vi "PXI_Host_LargeFXP_Write_NewMethod_Benchmark.vi"() -> ()   [LabVIEW 2018]
uses:
  <vilib>/Platform/TimedLoop/XDataNode/timing_clust.ctl
  <vilib>/Platform/TimedLoop/XDataNode/nitl_modes.ctl
  <vilib>/Platform/TimedLoop/XDataNode/wakeup.ctl
  cRIO RT/FPGA Bitfile Register Operations/Scalar IO Operations/TypeDefs/FXP Configuration.ctl
  <vilib>/fxp/LVFixedPointRepBitsTypeDef.ctl
  <vilib>/fxp/LVFixedPointRepRangeTypeDef.ctl
  cRIO RT/FPGA Bitfile Register Operations/Scalar IO Operations/Write Methods/Write Data Register/Instances/Write FXP.vi
  cRIO RT/FPGA Bitfile Register Operations/Scalar IO Operations/Write Methods/Write Data Register/Instances/Write U16.vi
  cRIO RT/FPGA Bitfile Register Operations/Scalar IO Operations/Write Methods/Write Data Register/Instances/Write U32.vi
  cRIO RT/FPGA Bitfile Register Operations/Scalar IO Operations/Write Methods/Write Data Register/Instances/Write U64.vi
  cRIO RT/FPGA Bitfile Register Operations/Scalar IO Operations/Write Methods/Write Data Register/Instances/Write U8.vi
  cRIO RT/FPGA Bitfile Register Operations/Scalar IO Operations/SubVIs/DBL to FXP Raw.vi
  cRIO RT/FPGA Bitfile Register Operations/Scalar IO Operations/Utilities/Find Register Offset.vi
  cRIO RT/FPGA Bitfile Register Operations/Scalar IO Operations/SubVIs/Check Register Data Store.vi
  cRIO RT/FPGA Bitfile Register Operations/Scalar IO Operations/Error Handling/Error 6001.vi
  cRIO RT/FPGA Bitfile Register Operations/Scalar IO Operations/Error Handling/Error 6000.vi
  cRIO RT/FPGA Bitfile Register Operations/Scalar IO Operations/Error Handling/Error 6002.vi
  cRIO RT/FPGA Bitfile Register Operations/Scalar IO Operations/Error Handling/Error 6006.vi
  <vilib>/FPGAPlugInAG/Dynamic/niLvFpga_Close_Dynamic.vi
  <vilib>/platform/TimedLoop/XDataNode/XDataNode.xnode
  <vilib>/rvi/interface/nirviCloseFPGA/nirviCloseFPGA.xnode
  cRIO RT/FPGA Bitfile Register Operations/Scalar IO Operations/FPGA Register IO.lvlib
  <vilib>/Platform/TimedLoop/XDataNode/XDNodeRunTimeDep.lvlib
panel:
  out "Maximum(s)":dbl
  out "Standard deviation":dbl
  out "Waveform Graph":dbl[](graph)
  out "error out":errorcluster
  out "Execution time (s)":dbl
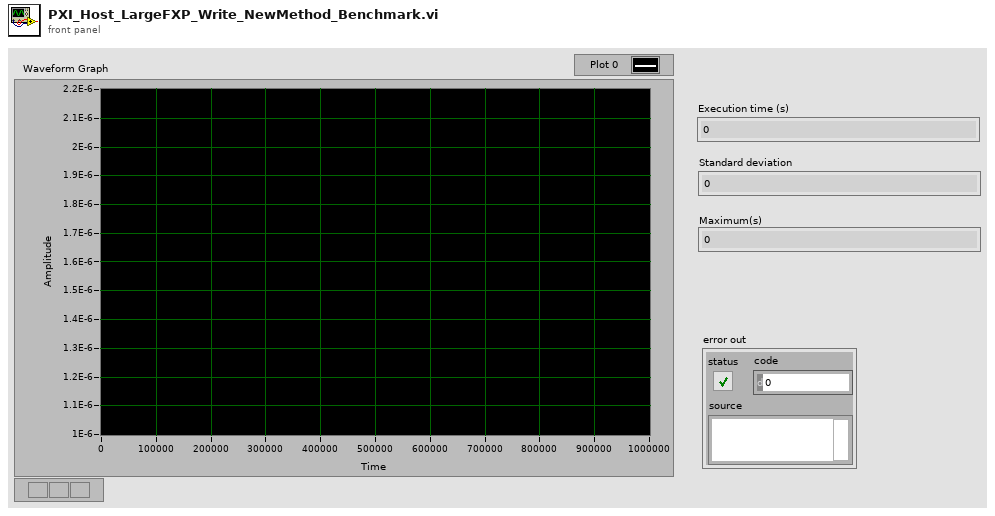
[diagram p1: front panel]
types:
  T1 = typedef "FPGA Register IO.lvlib/FXP Configuration.ctl" = cluster{"FXP Representation":T2, "FXP Range":T3}
  T2 = typedef "LVFixedPointRepBitsTypeDef.ctl" = cluster{"Signed":bool, "Word Length":u32, "Integer Word Length":i32}
  T3 = typedef "LVFixedPointRepRangeTypeDef.ctl" = cluster{"Range Min":dbl, "Range Max":dbl, "Delta":dbl}
  T4 = typedef "XDNodeRunTimeDep.lvlib/timing_clust.ctl" = cluster{"Expected End [f-1]":u64, "Actual End [f-1]":u64, "Finished Late? [f-1]":bool, "Expected End [i-1]":u64, "Actual End [i-1]":u64, "Finished Late? [i-1]":bool, "Expected Start [i]":u64, "Actual Start [i]":u64, "Expected Start [f]":u64, "Actual Start [f]":u64, "Source Name":string, "Structure Name":string, "Period":i64, "Deadline":i64, "Offset":i64, "Start":i64, "Priority":i32, "Timeout":i32, "Mode":T5, "Wakeup Reason":T6, "Error":errorcluster, "Source Type":string, "Secondary Source Type":string, "Global End Time":u64, "Global Start Time":u64, "Frame Duration":u64, "Iteration Duration":u64, "Assigned CPU":i32, "I/O Scan Engine Mode":u32}
  T5 = typedef "XDNodeRunTimeDep.lvlib/nitl_modes.ctl" = enum32{"No Change", "Process missed periods, maintain original phase", "Discard missed periods, maintain original phase", "Process missed periods, ignore original phase", "Discard missed periods, ignore original phase"}
  T6 = typedef "XDNodeRunTimeDep.lvlib/wakeup.ctl" = enum32{"Normal", "Aborted", "Asynchronous wakeup", "Timing source error", "Timed loop error", "Timeout"}
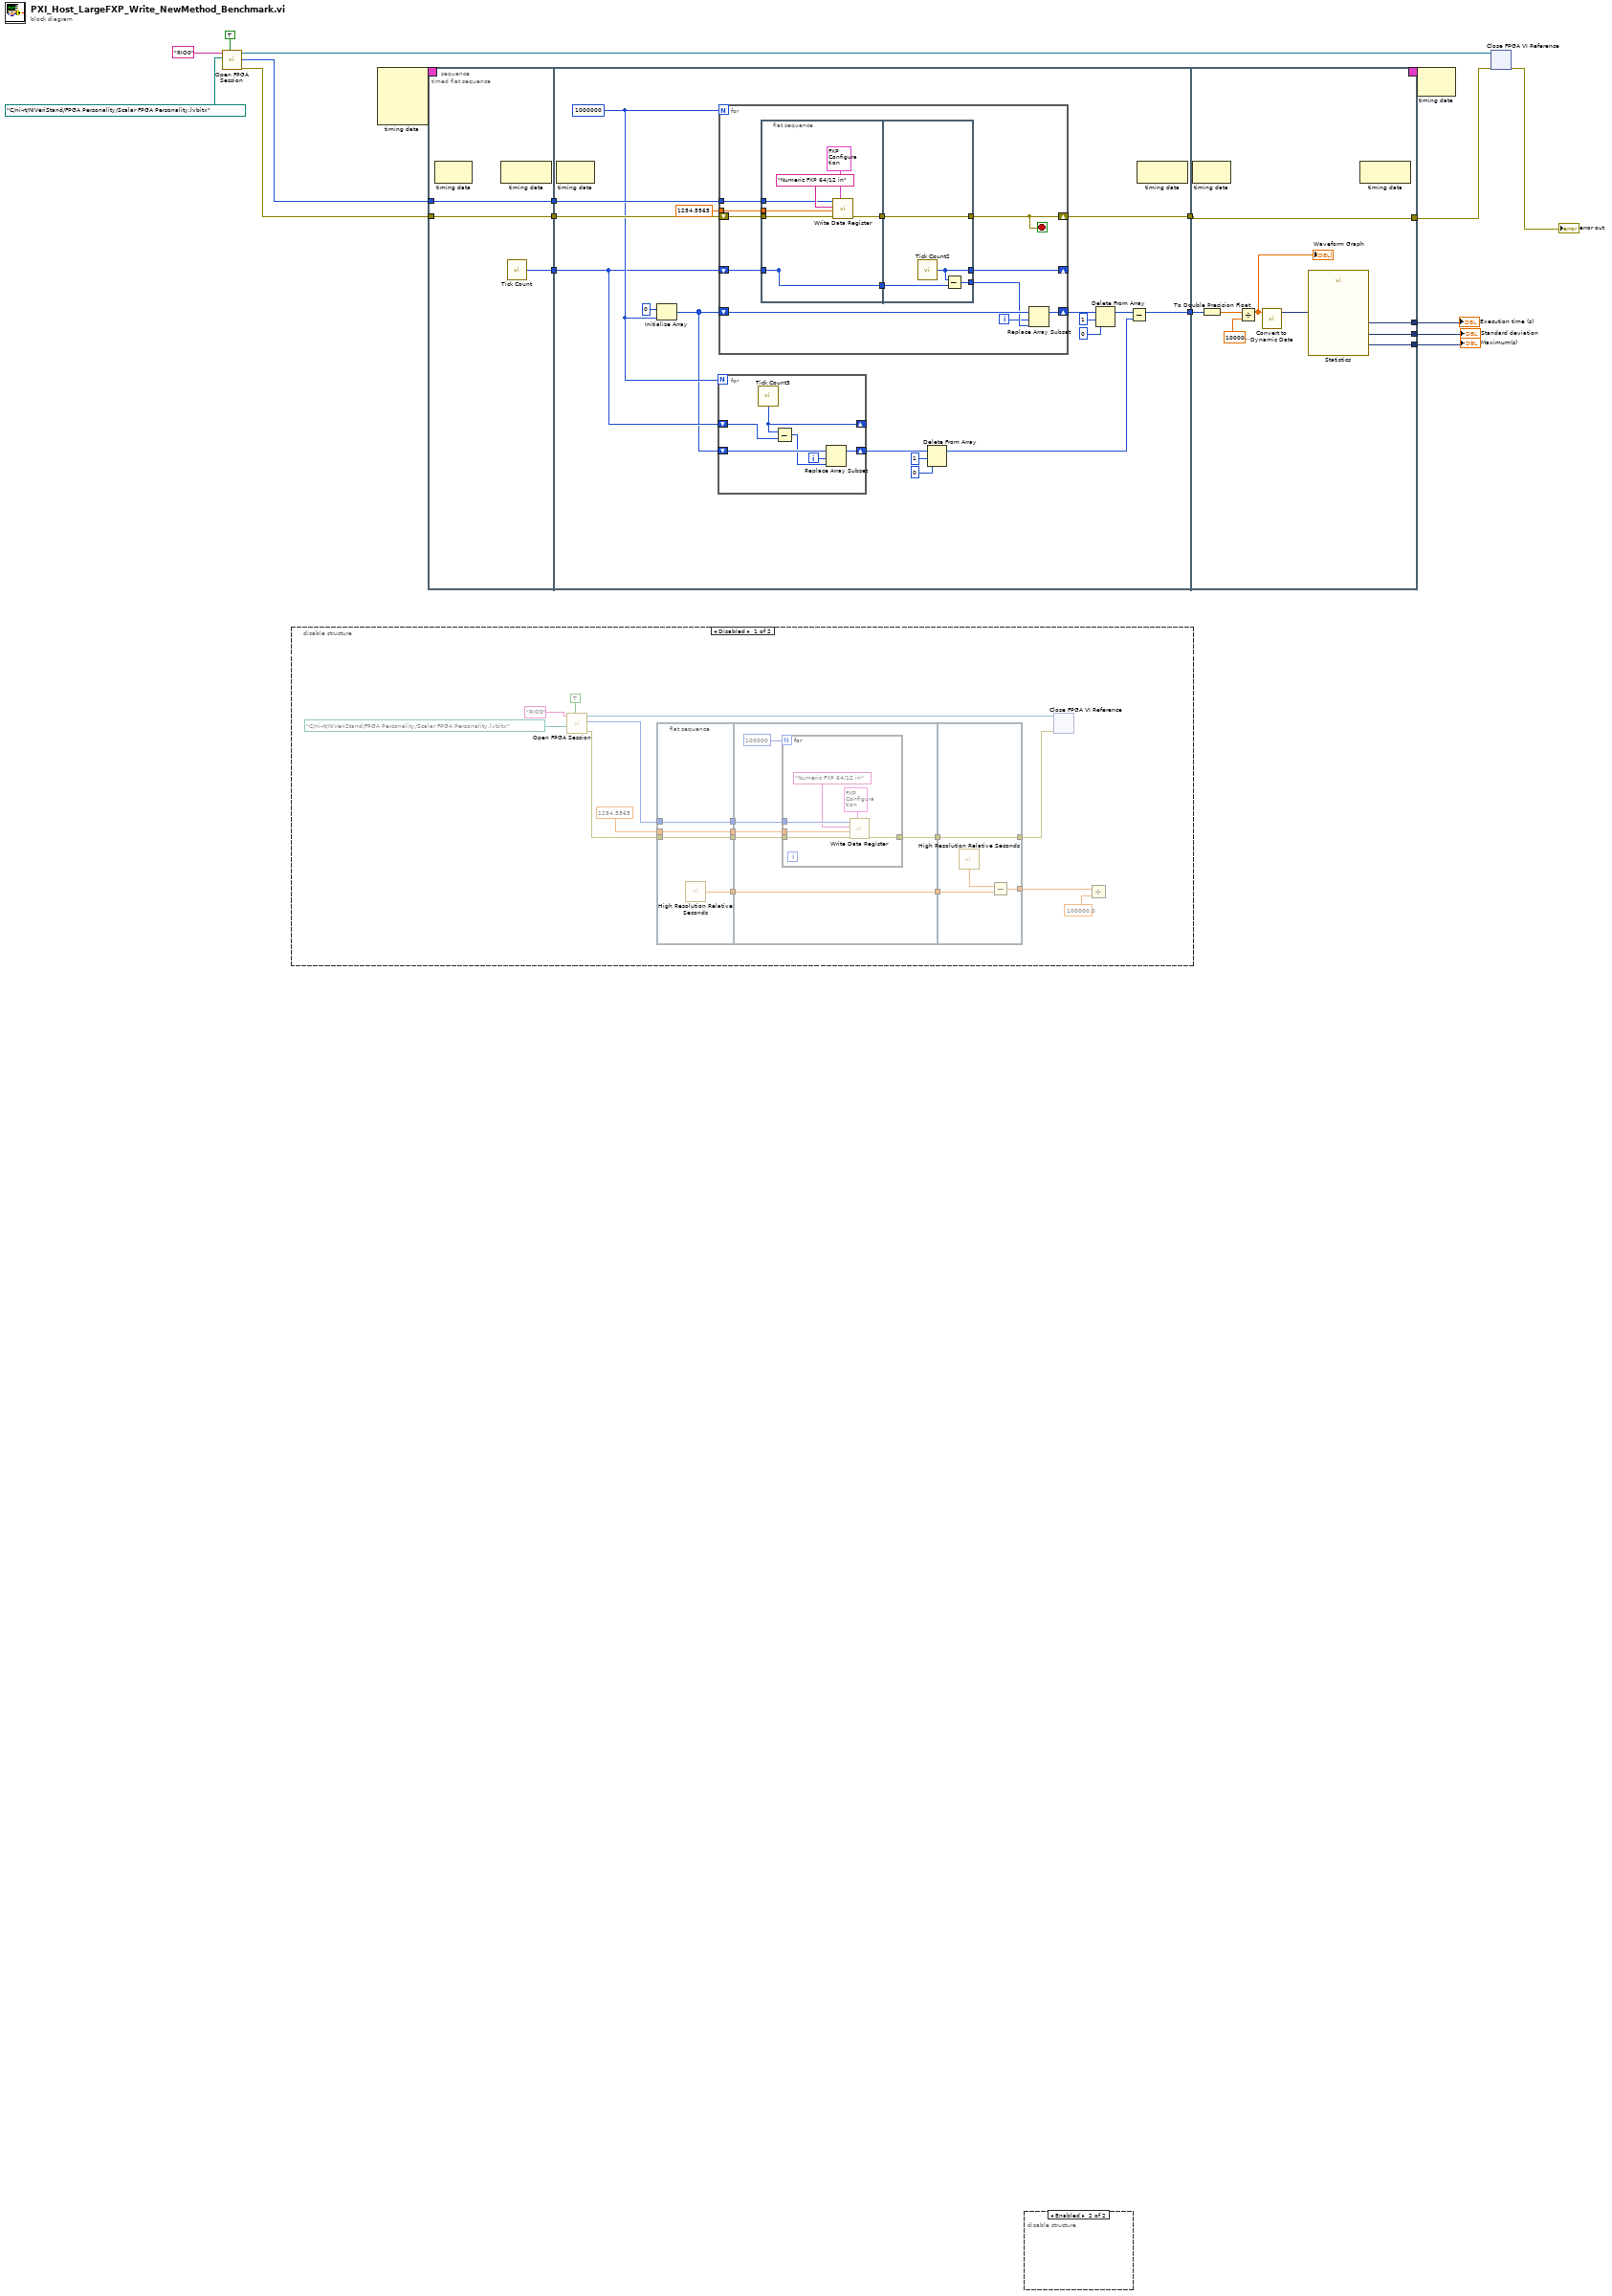
[diagram p0: block diagram]
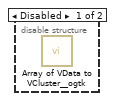
[diagram p3: hidden frame]
diagram:
  n1 = call "Open FPGA Session.vi"("run when loaded (T)"=TRUE, "bitfile path"=path "C:/ni-rt/NIVeriStand/FPGA Personality/Scalar FPGA Personality.lvbitx", "device address"="RIO0") -> ("error out"=w7:errorcluster, "session out"=w11:u32, "bitfile reference out"=w6:refnum<k20>)  [unwired: 6 in]
  n2 = disable-structure shown="Disabled" {
    frame Disabled {
      n3 = call "Open FPGA Session.vi"("run when loaded (T)"=TRUE, "bitfile path"=path "C:/ni-rt/NIVeriStand/FPGA Personality/Scalar FPGA Personality.lvbitx", "device address"="RIO0") -> ("error out"=w17:errorcluster, "session out"=w21:u32, "bitfile reference out"=w16:refnum<k20>)  [unwired: 6 in]
      n4 = flat-sequence {
        tunnel: [w33] -> w29
        tunnel: w21 -> [w32]
        tunnel: [w32] -> w28
        tunnel: w17 -> [w31]
        tunnel: [w31] -> w27
        tunnel: [w30] -> w26
        tunnel: 1254.5565 ("DBL Value") -> [w30]
        tunnel: [w38] -> w25
        tunnel: w29 -> [w38]
        tunnel: w28 -> [w37]
        tunnel: w27 -> [w36]
        tunnel: [w35] -> w24
        tunnel: w26 -> [w34]
        tunnel: w25 -> [w48]
        tunnel: [w47] -> w23
        tunnel: w24 -> [w46]
        tunnel: [w46] -> w15
        frame #0 {
          n5 = call <vilib>:"High Resolution Relative Seconds.vi"() -> ("relative seconds"=w33:dbl)
        }
        frame #1 {
          n6 = for {
            N: 100000 -> [_]
            tunnel: w37 -> [w43]
            tunnel: w36 -> [w45]
            tunnel: [w44] -> w35
            tunnel: w34 -> [w40]
            n7 = call-poly "Write Data Register.vi"("FXP Configuration"=T1 {"FXP Representation"={"Signed"=TRUE, "Word Length"=64, "Integer Word Length"=12}, "FXP Range"={"Range Min"=-2048.0, "Range Max"=2048.0, "Delta"=2.22045e-16}}, "error in"=w45, "DBL Value"=w40, "register name"="Numeric FXP 64/12 in", "session in"=w43) -> ("error out"=w44:errorcluster)  [unwired: 5 in, 1 out]
          }
        }
        frame #2 {
          n8 = call <vilib>:"High Resolution Relative Seconds.vi"() -> ("relative seconds"=w49:dbl)
          n9 = Subtract(x=w49, y=w48) -> (x-y=w47:dbl)
        }
      }
      n10 = xnode "Close FPGA VI Reference"("FPGA VI Reference In"=w16, "error in"=w15) -> ()  [unwired: 1 out]
      n11 = Divide(x=w23, y=100000.0) -> ()  [unwired: 1 out]
    }
    frame Enabled {
    }
  }
  n12 = node-c288() -> (w13:T4)  [unwired: 4 in]
  n13 = timed-sequence {
    timing: w13 -> [_]
    timing-out: [_] -> w12
    tunnel: w11 -> [w60]
    tunnel: w7 -> [w59]
    tunnel: [w55] -> w5
    tunnel: [w52] -> w3
    tunnel: [w51] -> w2
    tunnel: [w50] -> w1
    n14 = timed-flat-sequence {
      tunnel: w60 -> [w63]
      tunnel: [w63] -> w58
      tunnel: w59 -> [w62]
      tunnel: [w62] -> w57
      tunnel: [w61] -> w54
      tunnel: w58 -> [w82]
      tunnel: w57 -> [w81]
      tunnel: [w80] -> w56
      tunnel: w54 -> [w70]
      tunnel: [w67] -> w53
      tunnel: w56 -> [w122]
      tunnel: [w122] -> w55
      tunnel: w53 -> [w121]
      tunnel: [w119] -> w52
      tunnel: [w116] -> w51
      tunnel: [w115] -> w50
      frame #0 {
        n15 = node-c288() -> ()  [unwired: 1 in, 1 out]
        n16 = node-c288() -> ()  [unwired: 1 in, 1 out]
        n17 = call "Tick Count"() -> ("Tick Count(Ticks)"=w61:u32)
      }
      frame #1 {
        w71 = 1000000
        n18 = node-c288() -> ()  [unwired: 1 in, 1 out]
        n19 = Initialize Array(u32 0, w71) -> (w69:u32[])
        n20 = for {
          N: w71 -> [_]
          shift-right: [w83] -> w72
          shift-left: w69 -> [w86]
          shift-right: [w88] -> _
          shift-left: w70 -> [w87]
          i -> [w84]
          n21 = call "Tick Count3"() -> ("Tick Count(Ticks)"=w88:u32)
          n22 = Subtract(x=w88, y=w87) -> (x-y=w85:u32)
          n23 = Replace Array Subset(array=w86, new element=w85, index=w84) -> (w83:u32[])
        }
        n24 = for {
          N: w71 -> [_]
          tunnel: w82 -> [w101]
          shift-right: [w99] -> _
          shift-left: w70 -> [w98]
          shift-right: [w94] -> w78
          shift-left: w69 -> [w96]
          shift-right: [w92] -> w80
          shift-left: w81 -> [w102]
          tunnel: 1254.5565 ("DBL Value") -> [w91]
          i -> [w93]
          stop <- w92 stop-if-true
          n25 = flat-sequence {
            tunnel: w102 -> [w107]
            tunnel: w101 -> [w105]
            tunnel: [w106] -> w100
            tunnel: [w109] -> _
            tunnel: w98 -> [w109]
            tunnel: [w109] -> w97
            tunnel: w91 -> [w104]
            tunnel: [w113] -> w92
            tunnel: w100 -> [w113]
            tunnel: [w112] -> w99
            tunnel: w97 -> [w111]
            tunnel: [w110] -> w95
            frame #0 {
              n26 = call-poly "Write Data Register.vi"("FXP Configuration"=T1 {"FXP Representation"={"Signed"=TRUE, "Word Length"=64, "Integer Word Length"=12}, "FXP Range"={"Range Min"=-2048.0, "Range Max"=2048.0, "Delta"=2.22045e-16}}, "error in"=w107, "DBL Value"=w104, "register name"="Numeric FXP 64/12 in", "session in"=w105) -> ("error out"=w106:errorcluster)  [unwired: 5 in, 1 out]
            }
            frame #1 {
              n27 = call "Tick Count2"() -> ("Tick Count(Ticks)"=w112:u32)
              n28 = Subtract(x=w112, y=w111) -> (x-y=w110:u32)
            }
          }
          n29 = Replace Array Subset(array=w96, new element=w95, index=w93) -> (w94:u32[])
        }
        n30 = Delete From Array(array=w72, length=1, index=0) -> (array with subset deleted=w66:u32[])  [unwired: 1 out]
        n31 = Delete From Array(array=w78, length=1, index=0) -> (array with subset deleted=w68:u32[])  [unwired: 1 out]
        n32 = Subtract(x=w68, y=w66) -> (x-y=w67:u32[])
        n33 = node-c288() -> ()  [unwired: 1 in, 1 out]
      }
      frame #2 {
        n34 = node-c288() -> ()  [unwired: 1 in, 1 out]
        n35 = To Double Precision Float(number=w121) -> (double precision float=w118:dbl[])
        n36 = Divide(x=w118, y=1000000000.0) -> (x/y=w114:dbl[])
        "Waveform Graph" <- w114
        n37 = call "Convert to Dynamic Data"("Array"=w114) -> ("Dynamic Data Type"=w120:dynamicdata)  [unwired: 3 in]
        n38 = call "Statistics"("Signals"=w120) -> ("Standard Dev"=w116:dynamicdata, "Arithmetic Mean"=w119:dynamicdata, "Maximum"=w115:dynamicdata)  [unwired: 23 in, 1 out]
        n39 = node-c288() -> ()  [unwired: 1 in, 1 out]
      }
    }
  }
  "Execution time (s)" <- w3
  "Standard deviation" <- w2
  "Maximum(s)" <- w1
  n40 = disable-structure shown="Enabled" {
    frame Disabled {
      n41 = call <userlib>:"Array of VData to VCluster__ogtk.vi"() -> ()  [unwired: 10 in, 2 out]
    }
    frame Enabled {
    }
  }
  n42 = node-c288(w12) -> ()  [unwired: 1 out]
  n43 = xnode "Close FPGA VI Reference"("FPGA VI Reference In"=w6, "error in"=w5) -> ("error out"=→"error out":errorcluster)
